vi "dsf launch viewer property name.vi"() -> (3 "launch viewer property name":string)   [LabVIEW 2017, in "DSF Shared.lvlib"]
uses:
  Shared/DSF Shared.lvlib
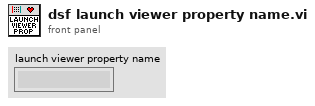
[diagram p1: front panel]
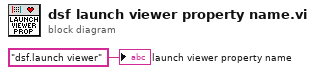
[diagram p0: block diagram]
diagram:
  "launch viewer property name" <- "dsf.launch viewer" ("Property Name")
